vi "Teleop.vi"(10 "Match Info":T1={"Autonomous Elapsed Seconds"=0.0, "TeleOp Elapsed Seconds"=0.0, "Disabled Elapsed Seconds"=0.0, "Visited Autonomous"=FALSE, "Visited TeleOp"=FALSE, "Visited Disabled"=FALSE, "Autonomous Settings"={"Autonomous Style"=enum."Independent", "VI Refnum"=refnum}}, 11 "Call Context":T2) -> ()   [LabVIEW 2015]
doc: "This VI is called for each TeleOp packet received from the DS where the robot is not disabled. It is often used to read from the joysticks and update I/O or to update setpoints for timed control loops. It should complete and return within 20 milliseconds or it may miss DS packets."
uses:
  <vilib>/Rock Robotics/WPI/DriverStation/WPI_DriverStationDerivedRobotMode.ctl
  <vilib>/Rock Robotics/WPI/DriverStation/WPI_DriverStationMatch Info.ctl
  Device Refnums.ctl
  Shooter Control.ctl
  Arm Mode TypeDef.ctl
  <vilib>/Rock Robotics/Network Tables/NT Read Number.vi
  Global Variables.vi
  <vilib>/Rock Robotics/Network Tables/NT Read Boolean.vi
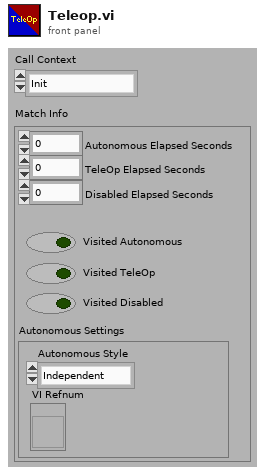
[diagram p1: front panel]
types:
  T1 = typedef "WPI_DriverStationMatch Info.ctl" = cluster{"Autonomous Elapsed Seconds":dbl, "TeleOp Elapsed Seconds":dbl, "Disabled Elapsed Seconds":dbl, "Visited Autonomous":bool, "Visited TeleOp":bool, "Visited Disabled":bool, "Autonomous Settings":cluster{"Autonomous Style":enum16{"Iterative", "Independent"}, "VI Refnum":refnum<vi>}}
  T2 = typedef "WPI_DriverStationDerivedRobotMode.ctl" = enum16{"Init", "Execute", "Stop"}
  T3 = typedef "Device Refnums.ctl" = string
  T4 = enum16{"Normal", "Make arm greater than override angle", "Make arm less than override angle"}
  T5 = typedef "Arm Mode TypeDef.ctl" = enum16{"Unknown", "Disabled", "Locked", "Shoot Batter", "Shoot Close", "Cross Defense", "Human Player Load", "Low Bar / Goal", "Manual"}
  T6 = typedef "WPI_EncoderDevRef.ctl" = cluster{"DevStatus":errorcluster, "EncoderIndex":T7, "CounterIndex":T8, "DistancePerCount":dbl, "Decoding Type":T9}
  T7 = typedef "FPGA_EncoderIdx.ctl" = enum8{"Enc 0", "Enc 1", "Enc 2", "Enc 3", "Enc 4", "Enc 5", "Enc 6", "Enc 7", "Invalid"}
  T8 = typedef "FPGA_CounterCtrSystemIndex.ctl" = enum8{"Ctr 0", "Ctr 1", "Ctr 2", "Ctr 3", "Ctr 4", "Ctr 5", "Ctr 6", "Ctr 7", "Invalid"}
  T9 = typedef "WPI_EncoderType.ctl" = enum16{"1x", "2x", "4x"}
  T10 = typedef "Switch_Input_TypeDef.ctl" = cluster{"SW 0":bool, "SW 1":bool, "SW 2":bool, "SW 3":bool, "SW 4":bool, "SW 5":bool, "SW 6":bool, "SW 7":bool, "SW 8":bool, "SW 9":bool, "SW 10":bool, "SW 11":bool, "SW 12":bool, "SW 13":bool, "SW 14":bool, "SW 15":bool}
  T11 = typedef "Logitech Attack 3 Button Map.ctl" = cluster{"Trigger Button 1":bool, "Thumb Button 2 ":bool, "Thumb Button 3":bool, "Thumb Button 4":bool, "Thumb Button 5":bool, "Bottom Button 6":bool, "Bottom Button 7":bool, "Bottom Button 8":bool, "Bottom Button 9":bool, "Bottom Button 10":bool, "Bottom Button 11":bool}
  T12 = typedef "Analog_Input_TypeDef.ctl" = cluster{"ANA 0":u8, "ANA 1":u8, "ANA 2":u8, "ANA 3":u8, "ANA 4":u8, "ANA 5":u8, "ANA 6":u8, "ANA 7":u8, "ANA 8":u8, "ANA 9":u8, "ANA 10":u8, "ANA 11":u8, "ANA 12":u8, "ANA 13":u8, "ANA 14":u8, "ANA 15":u8}
  T13 = typedef "Logitech Attack 3 Axis Map.ctl" = cluster{"X":dbl, "Y":dbl, "Throttle":dbl}
  T14 = typedef "Shooter Control.ctl" = cluster{"Fire":bool, "Open Claw":bool}
  T15 = typedef "WPI_MotorControlDeviceRef.ctl" = cluster{"DeviceStatus":errorcluster, "Type":T16, "PWM":cluster{"PWM Channel":T17, "DeadBand":T18}, "CAN":cluster{"Device Number":u8, "Control Mode":T19, "Semaphore":T20, "Max Vout":dbl, "TalonSRX Control Mode":T21}, "Invert":bool}
  T16 = typedef "WPI_MotorControlType.ctl" = enum16{"PWM", "CAN", "CANTalonSRX"}
  T17 = typedef "FPGA_DIOPWMChannel.ctl" = enum8{"PWM 0", "PWM 1", "PWM 2", "PWM 3", "PWM 4", "PWM 5", "PWM 6", "PWM 7", "PWM 8", "PWM 9", "PWM MXP 0", "PWM MXP 1", "PWM MXP 2", "PWM MXP 3", "PWM MXP 4", "PWM MXP 5", "PWM MXP 6", "PWM MXP 7", "PWM MXP 8", "PWM MXP 9", "Invalid"}
  T18 = typedef "WPI_PWMDeadband.ctl" = cluster{"Name":string, "maxPositivePwm":i32, "minPositivePwm":i32, "centerPwm":i32, "maxNegativePwm":i32, "minNegativePwm":i32, "angularRange":u16}
  T19 = typedef "WPI_CANJaguar_ControlMode.ctl" = enum8{"Percent VBus", "Current", "Speed", "Position", "Voltage"}
  T20 = typedef "Semaphore RefNum" = refnum<k1>
  T21 = typedef "WPI_CANTalonSRX_APIControlMode.ctl" = enum8{"Percent VBus", "Speed", "Position", "Slave", "Unchanged / Invalid", "Voltage Compensation", "Current", "Motion Profile"}
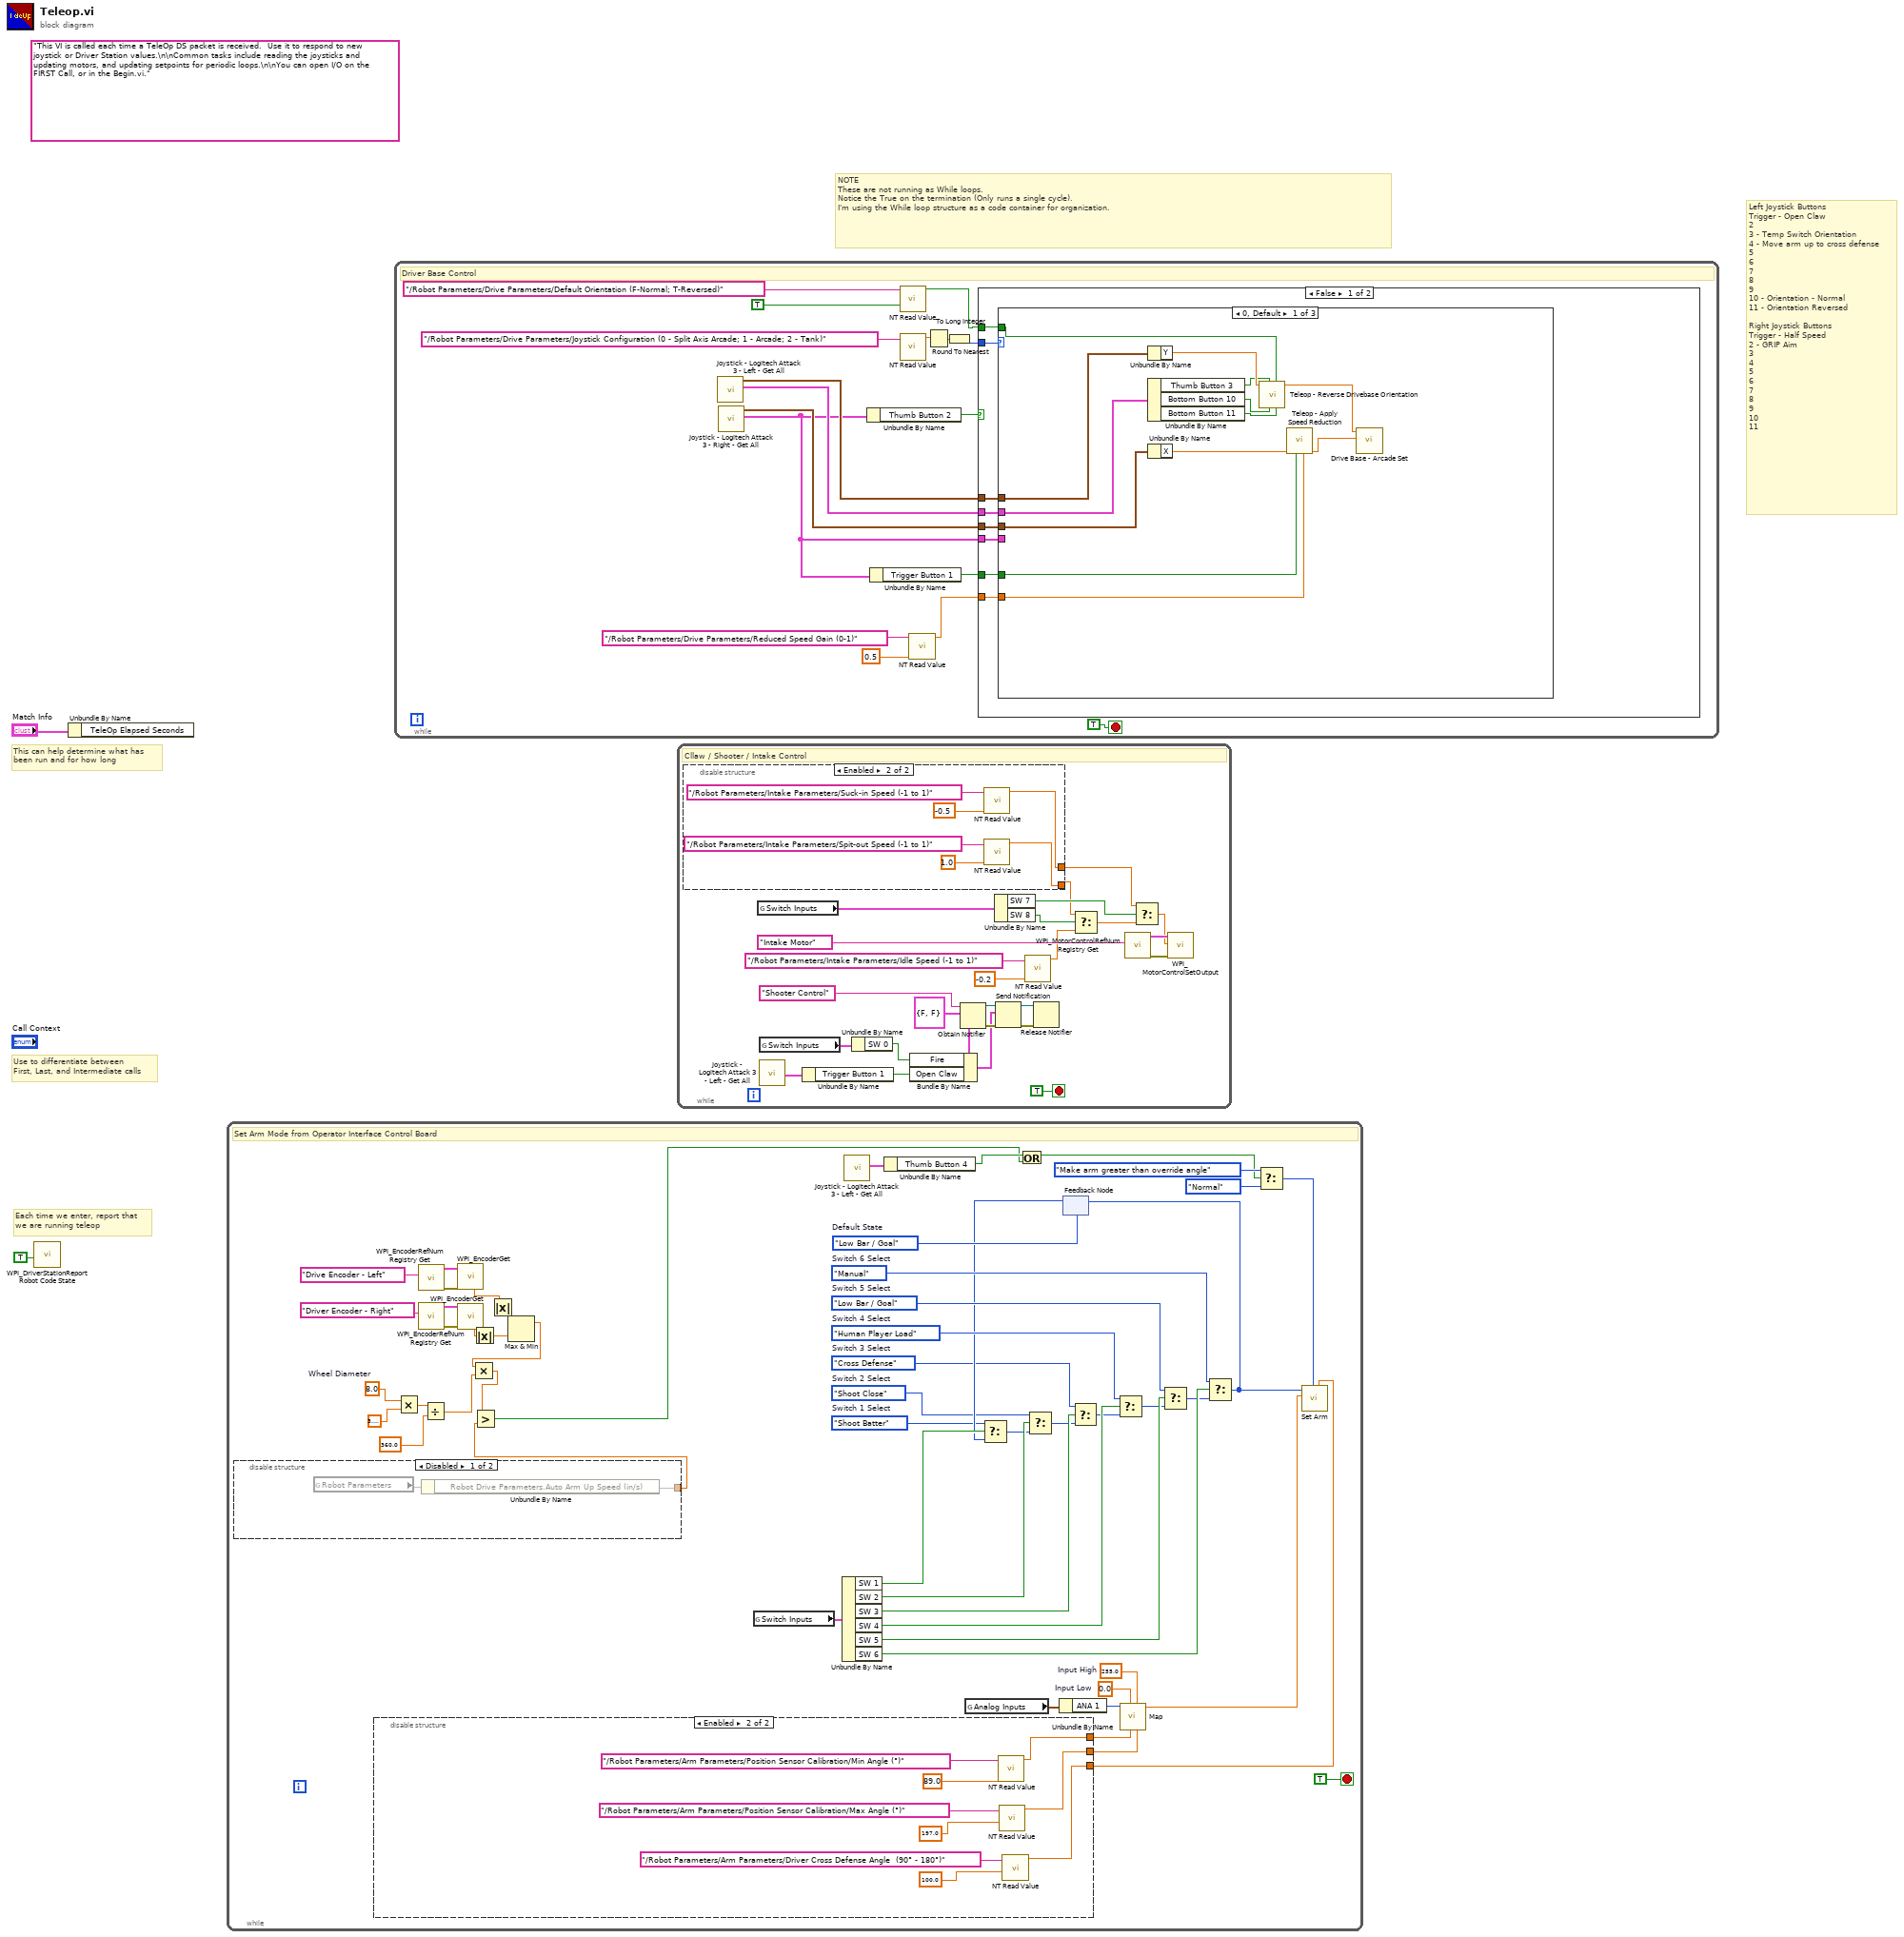
[diagram p0: block diagram]
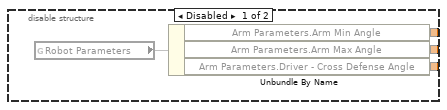
[diagram p2: hidden frame]
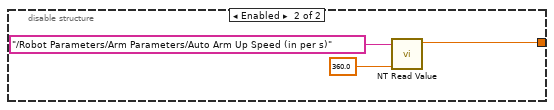
[diagram p3: hidden frame]
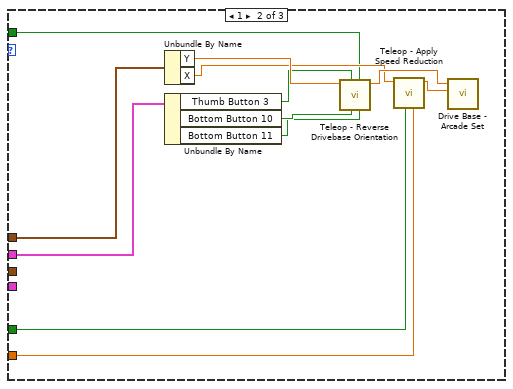
[diagram p4: hidden frame]
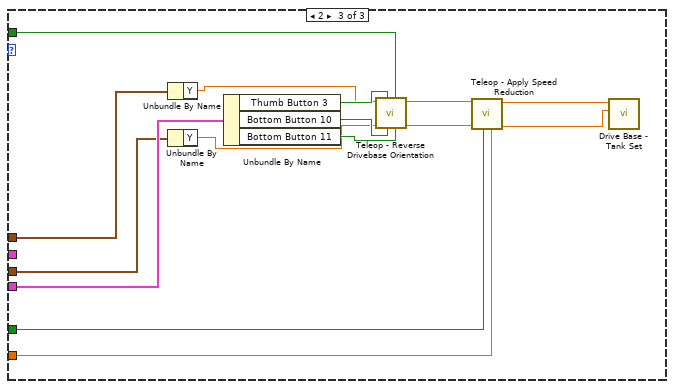
[diagram p5: hidden frame]
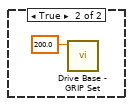
[diagram p6: hidden frame]
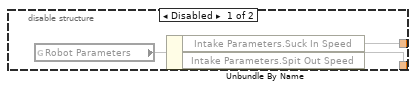
[diagram p7: hidden frame]
diagram:
  (unwired) "This VI is called each time a TeleOp DS packet is received.  Use it to respond to new joystick or Driver Station values.\n\nCommon tasks include reading the joysticks and updating motors, and updating setpoints for periodic loops.\n\nYou can open I/O on the FIRST Call, or in the Begin.vi."
  # "Left Joystick Buttons\nTrigger - Open Claw\n2\n3 - Temp Switch Orientation\n4 - Move arm up to cross defense\n5\n6\n7\n8\n9\n10 - Orientation - Normal\n11 - Orientation Reversed\n\nRight Joystick Buttons\nTrigger - Half Speed\n2 - GRIP Aim\n3\n4\n5\n6\n7\n8\n9\n10 \n11"
  # "NOTE\nThese are not running as While loops. \nNotice the True on the termination (Only runs a single cycle).\nI'm using the While loop structure as a code container for organization."
  # "Each time we enter, report that\nwe are running teleop"
  # "Use to differentiate between\nFirst, Last, and Intermediate calls"
  # "This can help determine what has\nbeen run and for how long"
  n1 = call <vilib>:"WPI_DriverStationReport Robot Code State.vi"("TeleOp"=TRUE ("Autonomous")) -> ()  [unwired: 10 in, 1 out]
  n2 = Unbundle By Name("Match Info") -> ()  [unwired: 1 out]
  n3 = while {
    stop <- TRUE stop-if-true
    w13 = 8.0  # Wheel Diameter
    w35 = 255.0  # Input High
    w34 = 0.0  # Input Low
    w39 = Arm_Mode_TypeDef."Shoot Batter"  # Switch 1 Select
    w38 = Arm_Mode_TypeDef."Shoot Close"  # Switch 2 Select
    w37 = Arm_Mode_TypeDef."Cross Defense"  # Switch 3 Select
    w46 = Arm_Mode_TypeDef."Low Bar / Goal"  # Switch 5 Select
    w53 = Arm_Mode_TypeDef."Low Bar / Goal"  # Default State
    w54 = Arm_Mode_TypeDef."Human Player Load"  # Switch 4 Select
    w55 = Arm_Mode_TypeDef."Manual"  # Switch 6 Select
    # "Set Arm Mode from Operator Interface Control Board"
    n4 = disable-structure shown="Disabled" {
      disable-tunnel: [w71 w74] -> w3
      frame Disabled {
        n5 = global read "Global Variables.vi" "Robot Parameters"() -> (w72)
        n6 = Unbundle By Name(w72) -> ("Robot Drive Parameters.Auto Arm Up Speed (in/s)"=w71)
      }
      frame Enabled {
        n7 = call-poly <vilib>:"NT Read Value.vi"("Default Value"=360.0, "Name"="/Robot Parameters/Arm Parameters/Auto Arm Up Speed (in per s)") -> ("Numeric"=w74:dbl)  [unwired: 8 in, 1 out]
      }
    }
    n8 = disable-structure shown="Enabled" {
      disable-tunnel: [w60 w69] -> w31
      disable-tunnel: [w59 w68] -> w30
      disable-tunnel: [w58 w67] -> w23
      frame Disabled {
        n9 = global read "Global Variables.vi" "Robot Parameters"() -> (w61)
        n10 = Unbundle By Name(w61) -> ("Arm Parameters.Arm Min Angle"=w60, "Arm Parameters.Arm Max Angle"=w59, "Arm Parameters.Driver - Cross Defense Angle"=w58)
      }
      frame Enabled {
        n11 = call-poly <vilib>:"NT Read Value.vi"("Default Value"=89.0, "Name"="/Robot Parameters/Arm Parameters/Position Sensor Calibration/Min Angle (°)") -> ("Numeric"=w69:dbl)  [unwired: 8 in, 1 out]
        n12 = call-poly <vilib>:"NT Read Value.vi"("Default Value"=197.0, "Name"="/Robot Parameters/Arm Parameters/Position Sensor Calibration/Max Angle (°)") -> ("Numeric"=w68:dbl)  [unwired: 8 in, 1 out]
        n13 = call-poly <vilib>:"NT Read Value.vi"("Default Value"=100.0, "Name"="/Robot Parameters/Arm Parameters/Driver Cross Defense Angle  (90° - 180°)") -> ("Numeric"=w67:dbl)  [unwired: 8 in, 1 out]
      }
    }
    n14 = Multiply(x=w13, y=3.141592653589793) -> (x*y=w12:dbl)
    n15 = call <vilib>:"WPI_EncoderRefNum Registry Get.vi"("refnum name"=T3 "Drive Encoder - Left" ("Device Name")) -> ("error out"=w21:errorcluster, "EncoderDevRef"=w20:T6)  [unwired: 9 in]
    n16 = call <vilib>:"WPI_EncoderRefNum Registry Get.vi"("refnum name"=T3 "Driver Encoder - Right" ("Device Name")) -> ("error out"=w19:errorcluster, "EncoderDevRef"=w18:T6)  [unwired: 9 in]
    n17 = Divide(x=w12, y=360.0) -> (x/y=w4:dbl)
    n18 = call <vilib>:"WPI_EncoderGet.vi"("error in (no error)"=w21, "EncoderDevRef"=w20) -> ("Rate"=w17:dbl)  [unwired: 4 in, 5 out]
    n19 = call <vilib>:"WPI_EncoderGet.vi"("error in (no error)"=w19, "EncoderDevRef"=w18) -> ("Rate"=w16:dbl)  [unwired: 4 in, 5 out]
    n20 = Absolute Value(x=w16) -> (abs(x)=w8:dbl)
    n21 = Absolute Value(x=w17) -> (abs(x)=w9:dbl)
    n22 = Max & Min(x=w9, y=w8) -> (max(x,y)=w10:dbl)  [unwired: 1 out]
    n23 = Multiply(x=w10, y=w4) -> (x*y=w5:dbl)
    n24 = Greater?(x=w5, y=w3) -> (0:w6:bool)
    n25 = global read "Global Variables.vi" "Switch Inputs"() -> (w57:T10)
    n26 = Unbundle By Name(w57) -> ("SW 1"=w49:bool, "SW 2"=w52:bool, "SW 3"=w51:bool, "SW 4"=w50:bool, "SW 5"=w45:bool, "SW 6"=w48:bool)
    n27 = call "Joystick - Logitech Attack 3 - Left - Get All.vi"() -> ("Buttons [Cluster]"=w28:T11)  [unwired: 7 in, 4 out]
    n28 = Unbundle By Name(w28) -> ("Thumb Button 4"=w24:bool)
    n29 = global read "Global Variables.vi" "Analog Inputs"() -> (w32:T12)
    n30 = Or(x=w24, y=w6) -> (x .or. y?=w7:bool)
    n31 = Unbundle By Name(w32) -> ("ANA 1"=w33:u8)
    n32 = feedback #1(w53) -> (w40:T5)
    n33 = Select(t=w39, s=w49, f=w40) -> (s? t:f=w41:T5)
    n34 = Select(t=w38, s=w52, f=w41) -> (s? t:f=w42:T5)
    n35 = Select(t=w37, s=w51, f=w42) -> (s? t:f=w43:T5)
    n36 = Select(t=w54, s=w50, f=w43) -> (s? t:f=w44:T5)
    n37 = call "Map.vi"("Output High"=w30, "Input High"=w35, "Output Low"=w31, "Input Low"=w34, "Input"=w33) -> ("Output"=w29:dbl)  [unwired: 6 in]
    n38 = Select(t=w46, s=w45, f=w44) -> (s? t:f=w47:T5)
    n39 = Select(t=w55, s=w48, f=w47) -> (s? t:f=w56:T5)
    n40 = feedback-in #1(w56) -> ()
    n41 = Select(t=T4."Make arm greater than override angle" ("Override Control"), s=w7, f=T4."Normal" ("Override Control")) -> (s? t:f=w25:T4)
    n42 = call "Set Arm.vi"("Override Angle"=w23, "Override Control"=w25, "Manual Arm Angle"=w29, "Arm Mode"=w56) -> ()  [unwired: 8 in]
  }
  n43 = while {
    stop <- TRUE stop-if-true
    # "Driver Base Control"
    n44 = call "Joystick - Logitech Attack 3 - Left - Get All.vi"() -> ("Buttons [Cluster]"=w89:T11, "Axes [Cluster]"=w88:T13)  [unwired: 7 in, 3 out]
    n45 = call "Joystick - Logitech Attack 3 - Right - Get All.vi"() -> ("Buttons [Cluster]"=w87:T11, "Axes [Cluster]"=w90:T13)  [unwired: 7 in, 3 out]
    n46 = Unbundle By Name(w87) -> ("Thumb Button 2"=w91:bool)
    n47 = Unbundle By Name(w87) -> ("Trigger Button 1"=w86:bool)
    n48 = call-poly <vilib>:"NT Read Value.vi"("Default Value"=TRUE ("Default Direction (F-Normal, T-Reversed)"), "Name"="/Robot Parameters/Drive Parameters/Default Orientation (F-Normal; T-Reversed)") -> ("Boolean"=w76:bool)  [unwired: 8 in, 1 out]
    n49 = call-poly <vilib>:"NT Read Value.vi"("Name"="/Robot Parameters/Drive Parameters/Joystick Configuration (0 - Split Axis Arcade; 1 - Arcade; 2 - Tank)") -> ("Numeric"=w82:dbl)  [unwired: 9 in, 1 out]
    n50 = call-poly <vilib>:"NT Read Value.vi"("Default Value"=0.5, "Name"="/Robot Parameters/Drive Parameters/Reduced Speed Gain (0-1)") -> ("Numeric"=w83:dbl)  [unwired: 8 in, 1 out]
    n51 = Round To Nearest(number=w82) -> (nearest integer value=w80:dbl)
    n52 = To Long Integer(number=w80) -> (32bit integer=w79:i32)
    n53 = case shown="False" w91 {
      tunnel: w79 -> [w100 _]
      tunnel: w83 -> [w99 _]
      tunnel: w87 -> [w98 _]
      tunnel: w90 -> [w97 _]
      tunnel: w89 -> [w96 _]
      tunnel: w88 -> [w95 _]
      tunnel: w86 -> [w94 _]
      tunnel: w76 -> [w93 _]
      frame False {
        n54 = case shown="0, Default" w100 {
          tunnel: w99 -> [w102 w118 w129]
          tunnel: w98 -> [_ _ w135]
          tunnel: w97 -> [w104 _ w134]
          tunnel: w96 -> [w105 w120 _]
          tunnel: w95 -> [w106 w119 w133]
          tunnel: w94 -> [w103 w117 w130]
          tunnel: w93 -> [w101 w114 w126]
          frame 0, Default {
            n55 = Unbundle By Name(w106) -> ("Y"=w113:dbl)
            n56 = Unbundle By Name(w105) -> ("Thumb Button 3"=w112:bool, "Bottom Button 10"=w111:bool, "Bottom Button 11"=w110:bool)
            n57 = Unbundle By Name(w104) -> ("X"=w108:dbl)
            n58 = call "Teleop - Reverse Drivebase Orientation.vi"("Reverse Orientation Switch (TB11)"=w110, "Default Direction (F-Normal, T-Reversed)"=w101, "Normal Orientation Switch (TB10)"=w111, "Momentary Flip (TB3)"=w112, "In 1"=w113) -> ("Out1"=w109:dbl)  [unwired: 5 in, 1 out]
            n59 = call "Teleop - Apply Speed Reduction.vi"("Gain"=w102, "Reduce Speed"=w103, "In 2"=w108) -> ("Out 2"=w107:dbl)  [unwired: 7 in, 1 out]
            n60 = call "Drive Base - Arcade Set.vi"("X"=w107, "Y"=w109) -> ()  [unwired: 9 in, 1 out]
          }
          frame 1 {
            n61 = Unbundle By Name(w119) -> ("Y"=w125:dbl, "X"=w115:dbl)
            n62 = Unbundle By Name(w120) -> ("Thumb Button 3"=w124:bool, "Bottom Button 10"=w123:bool, "Bottom Button 11"=w122:bool)
            n63 = call "Teleop - Reverse Drivebase Orientation.vi"("Reverse Orientation Switch (TB11)"=w122, "Default Direction (F-Normal, T-Reversed)"=w114, "Normal Orientation Switch (TB10)"=w123, "Momentary Flip (TB3)"=w124, "In 1"=w125) -> ("Out1"=w121:dbl)  [unwired: 5 in, 1 out]
            n64 = call "Teleop - Apply Speed Reduction.vi"("Gain"=w118, "Reduce Speed"=w117, "In 1"=w115) -> ("Out1"=w116:dbl)  [unwired: 7 in, 1 out]
            n65 = call "Drive Base - Arcade Set.vi"("X"=w116, "Y"=w121) -> ()  [unwired: 9 in, 1 out]
          }
          frame 2 {
            n66 = Unbundle By Name(w133) -> ("Y"=w137:dbl)
            n67 = Unbundle By Name(w134) -> ("Y"=w136:dbl)
            n68 = Unbundle By Name(w135) -> ("Thumb Button 3"=w140:bool, "Bottom Button 10"=w139:bool, "Bottom Button 11"=w138:bool)
            n69 = call "Teleop - Reverse Drivebase Orientation.vi"("Reverse Orientation Switch (TB11)"=w138, "Default Direction (F-Normal, T-Reversed)"=w126, "Normal Orientation Switch (TB10)"=w139, "Momentary Flip (TB3)"=w140, "In 2"=w136, "In 1"=w137) -> ("Out 2"=w131:dbl, "Out1"=w132:dbl)  [unwired: 4 in]
            n70 = call "Teleop - Apply Speed Reduction.vi"("Gain"=w129, "Reduce Speed"=w130, "In 2"=w131, "In 1"=w132) -> ("Out 2"=w127:dbl, "Out1"=w128:dbl)  [unwired: 6 in]
            n71 = call "Drive Base - Tank Set.vi"("Right"=w127, "Left"=w128) -> ()  [unwired: 9 in, 1 out]
          }
        }
      }
      frame True {
        n72 = call "Drive Base - GRIP Set.vi"("Target GRIP Area"=200.0) -> ()  [unwired: 10 in, 1 out]
      }
    }
  }
  n73 = while {
    stop <- TRUE stop-if-true
    w150 = T14 {"Fire"=FALSE, "Open Claw"=FALSE}
    # "Cllaw / Shooter / Intake Control"
    n74 = disable-structure shown="Enabled" {
      disable-tunnel: [w168 w170] -> w146
      disable-tunnel: [w167 w171] -> w145
      frame Disabled {
        n75 = global read "Global Variables.vi" "Robot Parameters"() -> (w169)
        n76 = Unbundle By Name(w169) -> ("Intake Parameters.Suck In Speed"=w168, "Intake Parameters.Spit Out Speed"=w167)
      }
      frame Enabled {
        n77 = call-poly <vilib>:"NT Read Value.vi"("Default Value"=-0.5, "Name"="/Robot Parameters/Intake Parameters/Suck-in Speed (-1 to 1)") -> ("Numeric"=w170:dbl)  [unwired: 8 in, 1 out]
        n78 = call-poly <vilib>:"NT Read Value.vi"("Default Value"=1.0, "Name"="/Robot Parameters/Intake Parameters/Spit-out Speed (-1 to 1)") -> ("Numeric"=w171:dbl)  [unwired: 8 in, 1 out]
      }
    }
    n79 = global read "Global Variables.vi" "Switch Inputs"() -> (w156:T10)
    n80 = global read "Global Variables.vi" "Switch Inputs"() -> (w166:T10)
    n81 = call "Joystick - Logitech Attack 3 - Left - Get All.vi"() -> ("Buttons [Cluster]"=w164:T11)  [unwired: 7 in, 4 out]
    n82 = Unbundle By Name(w164) -> ("Trigger Button 1"=w148:bool)
    n83 = Unbundle By Name(w166) -> ("SW 0"=w147:bool)
    n84 = Bundle By Name(cluster=w150, "Fire"=w147, "Open Claw"=w148) -> (w149:T14)
    n85 = Obtain Notifier(name (unnamed)="Shooter Control", notification data type=w150) -> (notifier out=w151:refnum<notifier>, error out=w152:errorcluster)  [unwired: 2 in, 1 out]
    n86 = Unbundle By Name(w156) -> ("SW 7"=w162:bool, "SW 8"=w161:bool)
    n87 = Send Notification(notification=w149, notifier=w151, error in (no error)=w152) -> (notifier out=w154:refnum<notifier>, error out=w153:errorcluster)
    n88 = call-poly <vilib>:"NT Read Value.vi"("Default Value"=-0.2, "Name"="/Robot Parameters/Intake Parameters/Idle Speed (-1 to 1)") -> ("Numeric"=w142:dbl)  [unwired: 8 in, 1 out]
    n89 = Release Notifier(notifier=w154, error in (no error)=w153) -> ()  [unwired: 1 in, 3 out]
    n90 = Select(t=w145, s=w161, f=w142) -> (s? t:f=w163:dbl)
    n91 = call <vilib>:"WPI_MotorControlRefNum Registry Get.vi"("refnum name"=T3 "Intake Motor" ("Device Name")) -> ("error out"=w159:errorcluster, "MotorControlDevRef"=w160:T15)  [unwired: 9 in]
    n92 = Select(t=w146, s=w162, f=w163) -> (s? t:f=w157:dbl)
    n93 = call <vilib>:"WPI_MotorControlSetOutput.vi"("error in (no error)"=w159, "Output"=w157, "MotorControlDevRef"=w160) -> ()  [unwired: 6 in, 3 out]
  }
